vi "PFD_Attitude.vi"(8 "Refresh Rate (Hz)":u32=60) -> ()   [LabVIEW 2023]
uses:
  <vilib>/Utility/miscctls.llb/LVBoundsTypeDef.ctl
  PFD_global.vi
panel:
  in  "Draw Area Size":T1={"Width"=500, "Height"=500}
  in  "att_center":cluster{"y":i16, "y":i16}={"y"=250, "y"=250}
  out "att_pitch":i16
  out "att_roll":i16
  out "x .or. y?":bool
  out "PFD_AttitudeControl":cluster{"Roll":sgl, "Pitch":sgl}
  out "PFD_Attitude":picture
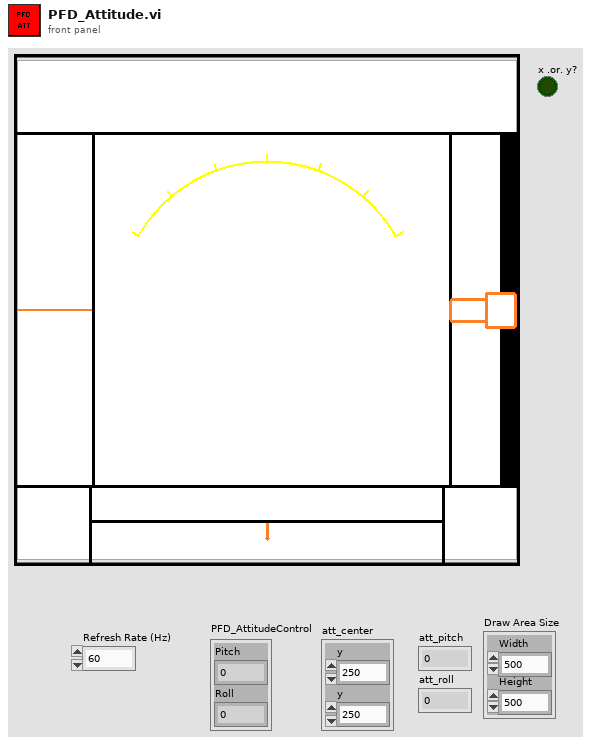
[diagram p1: front panel]
types:
  T1 = typedef "LVBoundsTypeDef.ctl" = cluster{"Width":u32, "Height":u32}
  T2 = cluster{"left":i16, "top":i16, "right":i16, "bottom":i16}
  T3 = cluster{"Width":u16, "Style":enum32{"Solid", "Dash", "Dot", "DashDot", "DashDotDot"}}
  T4 = cluster{"Font Name:":string, "Size":i16, "Strikeout?":bool, "Italic?":bool, "Underline?":bool, "Outline?":bool, "Shadow?":bool, "Bold?":bool}
  T5 = enum16{"User-specified Font", "Application Font", "System Font", "Dialog Font"}
  T6 = cluster{"horizontal":enum16{"left", "center", "right"}, "vertical":enum16{"top", "center", "bottom"}}
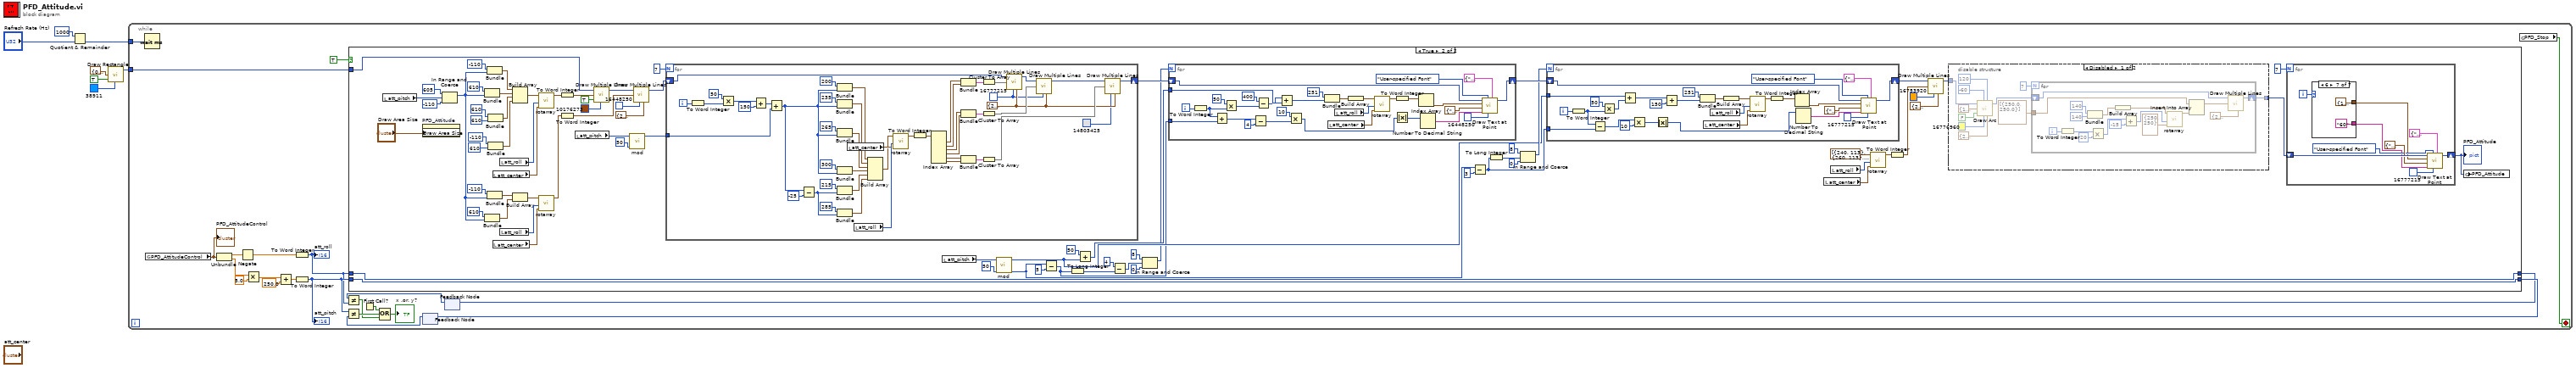
[diagram p0: block diagram]
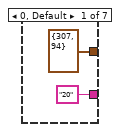
[diagram p3: hidden frame]
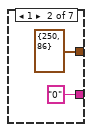
[diagram p4: hidden frame]
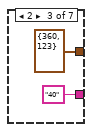
[diagram p5: hidden frame]
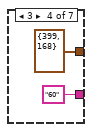
[diagram p6: hidden frame]
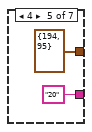
[diagram p7: hidden frame]
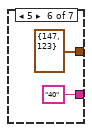
[diagram p8: hidden frame]
diagram:
  n1 = Quotient & Remainder(x=u32 1000, y="Refresh Rate (Hz)") -> (floor(x/y)=w2:u32)  [unwired: 1 out]
  n2 = call <vilib>:"Draw Rectangle.vi"("rect"=T2 {"left"=0, "top"=0, "right"=500, "bottom"=500}, "fill?(F)"=TRUE, "color(black)"=u32 38911 ("Air Color")) -> ("new picture"=w5:picture)  [unwired: 6 in]
  n3 = while {
    tunnel: w5 -> [w29]
    tunnel: w2 -> [w17]
    stop <- w8 stop-if-true
    n4 = Wait (ms)(milliseconds to wait=w17) -> ()  [unwired: 1 out]
    n5 = global read "PFD_global.vi" "PFD_AttitudeControl"() -> (w16:cluster{"Roll":sgl, "Pitch":sgl})
    "PFD_AttitudeControl" <- w16
    n6 = Unbundle(w16) -> ("Roll"=w15:sgl, "Pitch"=w27:sgl)
    n7 = Negate(x=w15) -> (-x=w14:sgl)
    n8 = Multiply(x=w27, y=sgl 5.0) -> (x*y=w13:sgl)
    n9 = Add(x=w13, y=sgl 250.0) -> (x+y=w25:sgl)
    n10 = To Word Integer(number=w14) -> (16bit integer=w11:i16)
    "att_roll" <- w11
    n11 = To Word Integer(number=w25) -> (16bit integer=w12:i16)
    "att_pitch" <- w12
    n12 = case shown="True" TRUE {
      tunnel: w29 -> [_ w107]
      tunnel: w11 -> [w30 w101]
      tunnel: w12 -> [w31 w102]
      tunnel: [w31 w102] -> w23
      tunnel: [w30 w101] -> w20
      frame False {
      }
      frame True {
        n13 = local read "att_pitch"() -> (w76:i16)
        n14 = property on="PFD_Attitude" class="Pict"("Draw Area Size"="Draw Area Size") -> ()  [unwired: 2 in, 2 out]
        n15 = In Range and Coerce(upper limit=i16 605, x=w76, lower limit=i16 -110) -> (coerced(x)=w73:i16)  [unwired: 1 out]
        n16 = Bundle(i16 610, "upper limit"=w73) -> (w64:cluster{i16, "upper limit":i16})  [unwired: 1 in]
        n17 = Bundle(i16 610, "upper limit"=w73) -> (w54:cluster{i16, "upper limit":i16})  [unwired: 1 in]
        n18 = Bundle(i16 -110, "upper limit"=w73) -> (w63:cluster{i16, "upper limit":i16})  [unwired: 1 in]
        n19 = Bundle(i16 -110, "upper limit"=w73) -> (w53:cluster{i16, "upper limit":i16})  [unwired: 1 in]
        n20 = Bundle(i16 610, i16 610) -> (w65:cluster{i16, i16})  [unwired: 1 in]
        n21 = Bundle(i16 -110, i16 610) -> (w66:cluster{i16, i16})  [unwired: 1 in]
        n22 = local read "att_center"() -> (w68:cluster{"y":i16, "y":i16})
        n23 = local read "att_center"() -> (w52:cluster{"y":i16, "y":i16})
        n24 = local read "att_roll"() -> (w67:i16)
        n25 = local read "att_roll"() -> (w51:i16)
        n26 = Build Array(w63, w64, w65, w66) -> (w56:cluster{i16, "upper limit":i16}[])
        n27 = Build Array(w53, w54) -> (w55:cluster{i16, "upper limit":i16}[])
        n28 = call "rotarray.vi"("Pixel Center"=w68, "Angle"=w67, "Array in"=w56) -> ("Array out"=w71:cluster{dbl, dbl}[])  [unwired: 8 in]
        n29 = call "rotarray.vi"("Pixel Center"=w52, "Angle"=w51, "Array in"=w55) -> ("Array out"=w47:cluster{dbl, dbl}[])  [unwired: 8 in]
        n30 = To Word Integer(number=w71) -> (16bit integer=w72:cluster{i16, i16}[])
        n31 = To Word Integer(number=w47) -> (16bit integer=w48:cluster{i16, i16}[])
        n32 = local read "att_pitch"() -> (w78:i16)
        n33 = call <vilib>:"Draw Multiple Lines.vi"("picture"=w107, "line endpoints"=w72, "fill?(F)"=TRUE, "color(black)"=u32 10176273 ("Ground Color")) -> ("new picture"=w46:picture)  [unwired: 5 in]
        n34 = call "mod.vi"("Divide"=i16 50, "Value In"=w78) -> ("Value out"=w104:i16)  [unwired: 8 in, 1 out]
        n35 = call <vilib>:"Draw Multiple Lines.vi"("picture"=w46, "line endpoints"=w48, "color(black)"=u32 16448250, "pen"=T3 {"Width"=2, "Style"=enum."Solid"}) -> ("new picture"=w77:picture)  [unwired: 5 in]
        n36 = for {
          N: 7 ("Numeric") -> [_]
          shift-right: [w239] -> w103
          shift-left: w77 -> [w263]
          tunnel: w104 -> [w251]
          i -> [w259]
          w237 = u32 16777215 ("color(black)")
          w245 = T3 {"Width"=2, "Style"=enum."Solid"} ("pen")
          n37 = To Word Integer(number=w259) -> (16bit integer=w255:i16)
          n38 = Multiply(x=i16 50, y=w255) -> (x*y=w219:i16)
          n39 = Add(x=w219, y=i16 150) -> (x+y=w218:i16)
          n40 = Add(x=w218, y=w251) -> (x+y=w243:i16)
          n41 = Subtract(x=w243, y=i16 -25 ("y 2")) -> (x-y=w241:i16)
          n42 = Bundle(i16 200, w243) -> (w227:cluster{i16, i16})  [unwired: 1 in]
          n43 = Bundle(i16 235, w243) -> (w226:cluster{i16, i16})  [unwired: 1 in]
          n44 = Bundle(i16 265, w243) -> (w225:cluster{i16, i16})  [unwired: 1 in]
          n45 = Bundle(i16 300, w243) -> (w224:cluster{i16, i16})  [unwired: 1 in]
          n46 = Bundle("Numeric 2"=i16 215, w241) -> (w223:cluster{"Numeric 2":i16, i16})  [unwired: 1 in]
          n47 = Bundle("Numeric 3"=i16 285, w241) -> (w222:cluster{"Numeric 3":i16, i16})  [unwired: 1 in]
          n48 = local read "att_center"() -> (w235:cluster{"y":i16, "y":i16})
          n49 = local read "att_roll"() -> (w236:i16)
          n50 = Build Array(w227, w226, w225, w224, w223, w222) -> (w221:cluster{"Numeric 3":i16, i16}[])
          n51 = call "rotarray.vi"("Pixel Center"=w235, "Angle"=w236, "Array in"=w221) -> ("Array out"=w252:cluster{dbl, dbl}[])  [unwired: 8 in]
          n52 = To Word Integer(number=w252) -> (16bit integer=w234:cluster{i16, i16}[])
          n53 = Index Array(array=w234) -> (element #1=w233:cluster{i16, i16}, element #2=w232:cluster{i16, i16}, element #3=w231:cluster{i16, i16}, element #4=w230:cluster{i16, i16}, element #5=w229:cluster{i16, i16}, element #6=w228:cluster{i16, i16})  [unwired: 6 in]
          n54 = Bundle(w233, w232) -> (w250:cluster{cluster{i16, i16}, cluster{i16, i16}})  [unwired: 1 in]
          n55 = Bundle(w231, w230) -> (w249:cluster{cluster{i16, i16}, cluster{i16, i16}})  [unwired: 1 in]
          n56 = Bundle(w229, w228) -> (w238:cluster{cluster{i16, i16}, cluster{i16, i16}})  [unwired: 1 in]
          n57 = Cluster To Array(cluster=w250) -> (array=w254:cluster{i16, i16}[])
          n58 = Cluster To Array(cluster=w249) -> (array=w253:cluster{i16, i16}[])
          n59 = Cluster To Array(cluster=w238) -> (array=w246:cluster{i16, i16}[])
          n60 = call <vilib>:"Draw Multiple Lines.vi"("picture"=w263, "line endpoints"=w254, "color(black)"=w237, "pen"=w245) -> ("new picture"=w256:picture)  [unwired: 5 in]
          n61 = call <vilib>:"Draw Multiple Lines.vi"("picture"=w256, "line endpoints"=w253, "color(black)"=w237, "pen"=w245) -> ("new picture"=w247:picture)  [unwired: 5 in]
          n62 = call <vilib>:"Draw Multiple Lines.vi"("picture"=w247, "line endpoints"=w246, "color(black)"=u32 14803425, "pen"=w245) -> ("new picture"=w239:picture)  [unwired: 5 in]
        }
        n63 = local read "att_pitch"() -> (w94:i16)
        n64 = call "mod.vi"("Divide"=i16 50, "Value In"=w94) -> ("Ceil"=w81:i16, "Value out"=w91:i16)  [unwired: 8 in]
        n65 = Subtract(x=w81, y=i16 5) -> (x-y=w82:i16)
        n66 = To Long Integer(number=w82) -> (32bit integer=w83:i32)
        n67 = Add(x=i16 50 ("y"), y=w91) -> (x+y=w90:i16)
        n68 = Subtract(x=4 ("Numeric"), y=w83) -> (x-y=w85:i32)
        n69 = In Range and Coerce(upper limit=8, x=w85, lower limit=0) -> (coerced(x)=w84:i32)  [unwired: 1 out]
        n70 = for {
          N: w84 -> [_]
          shift-right: [w205] -> w100
          shift-left: w103 -> [w207]
          tunnel: w90 -> [w198]
          tunnel: w82 -> [w191]
          i -> [w201]
          n71 = To Word Integer(number=w201) -> (16bit integer=w192:i16)
          n72 = Add(x=w192, y=w191) -> (x+y=w190:i16)
          n73 = Multiply(x=i16 50, y=w192) -> (x*y=w197:i16)
          n74 = Subtract(x=w190, y=i16 4 ("y 2")) -> (x-y=w188:i16)
          n75 = Subtract(x=i16 400 ("y 4"), y=w197) -> (x-y=w196:i16)
          n76 = Add(x=w196, y=w198) -> (x+y=w195:i16)
          n77 = Multiply(x=i16 10, y=w188) -> (x*y=w193:i16)
          n78 = Bundle("Numeric 2"=i16 251, w195) -> (w212:cluster{"Numeric 2":i16, i16})  [unwired: 1 in]
          n79 = local read "att_center"() -> (w203:cluster{"y":i16, "y":i16})
          n80 = local read "att_roll"() -> (w206:i16)
          n81 = Build Array(w212) -> (w211:cluster{"Numeric 2":i16, i16}[])
          n82 = call "rotarray.vi"("Pixel Center"=w203, "Angle"=w206, "Array in"=w211) -> ("Array out"=w209:cluster{dbl, dbl}[])  [unwired: 8 in]
          n83 = To Word Integer(number=w209) -> (16bit integer=w208:cluster{i16, i16}[])
          n84 = Absolute Value(x=w193) -> (abs(x)=w202:i16)
          n85 = Index Array(array=w208) -> (element=w210:cluster{i16, i16})  [unwired: 1 in]
          n86 = Number To Decimal String(number=w202) -> (decimal integer string=w214:string)  [unwired: 1 in]
          n87 = call <vilib>:"Draw Text at Point.vi"("[user-specified font]"=T4 {"Font Name:"="a", "Size"=18, "Strikeout?"=FALSE, "Italic?"=FALSE, "Underline?"=FALSE, "Outline?"=FALSE, "Shadow?"=FALSE, "Bold?"=TRUE}, "text color(black)"=u32 16448250, "desired font(Application)"=T5."User-specified Font", "text"=w214, "alignment(left, top)"=T6 {"horizontal"=enum."center", "vertical"=enum."center"}, "origin"=w210, "picture"=w207) -> ("new picture"=w205:picture)  [unwired: 3 in, 1 out]
        }
        n88 = Subtract(x=w81, y=i16 3) -> (x-y=w80:i16)
        n89 = To Long Integer(number=w80) -> (32bit integer=w98:i32)
        n90 = In Range and Coerce(upper limit=8, x=w98, lower limit=0) -> (coerced(x)=w95:i32)  [unwired: 1 out]
        n91 = for {
          N: w95 -> [_]
          shift-right: [w173] -> w33
          shift-left: w100 -> [w172]
          tunnel: w91 -> [w168]
          tunnel: w80 -> [w160]
          i -> [w185]
          n92 = To Word Integer(number=w185) -> (16bit integer=w161:i16)
          n93 = Subtract(x=w161, y=w160) -> (x-y=w163:i16)
          n94 = Multiply(x=i16 50, y=w161) -> (x*y=w183:i16)
          n95 = Add(x=w168, y=w183) -> (x+y=w167:i16)
          n96 = Multiply(x=w163, y=i16 10) -> (x*y=w162:i16)
          n97 = Absolute Value(x=w162) -> (abs(x)=w187:i16)
          n98 = Add(x=w167, y=i16 150) -> (x+y=w165:i16)
          n99 = Bundle("Numeric 2"=i16 251, w165) -> (w178:cluster{"Numeric 2":i16, i16})  [unwired: 1 in]
          n100 = local read "att_center"() -> (w169:cluster{"y":i16, "y":i16})
          n101 = local read "att_roll"() -> (w171:i16)
          n102 = Build Array(w178) -> (w177:cluster{"Numeric 2":i16, i16}[])
          n103 = call "rotarray.vi"("Pixel Center"=w169, "Angle"=w171, "Array in"=w177) -> ("Array out"=w175:cluster{dbl, dbl}[])  [unwired: 8 in]
          n104 = To Word Integer(number=w175) -> (16bit integer=w176:cluster{i16, i16}[])
          n105 = Index Array(array=w176) -> (element=w174:cluster{i16, i16})  [unwired: 1 in]
          n106 = Number To Decimal String(number=w187) -> (decimal integer string=w186:string)  [unwired: 1 in]
          n107 = call <vilib>:"Draw Text at Point.vi"("[user-specified font]"=T4 {"Font Name:"="a", "Size"=18, "Strikeout?"=FALSE, "Italic?"=FALSE, "Underline?"=FALSE, "Outline?"=FALSE, "Shadow?"=FALSE, "Bold?"=TRUE}, "text color(black)"=u32 16777215, "desired font(Application)"=T5."User-specified Font", "text"=w186, "alignment(left, top)"=T6 {"horizontal"=enum."center", "vertical"=enum."center"}, "origin"=w174, "picture"=w172) -> ("new picture"=w173:picture)  [unwired: 3 in, 1 out]
        }
        n108 = local read "att_center"() -> (w37:cluster{"y":i16, "y":i16})
        n109 = local read "att_roll"() -> (w36:i16)
        n110 = call "rotarray.vi"("Pixel Center"=w37, "Angle"=w36, "Array in"=cluster{"x":i16, "y":i16}[] [{"x"=240, "y"=113}, {"x"=260, "y"=113}, {"x"=250, "y"=103}, {"x"=240, "y"=113}] ("line endpoints")) -> ("Array out"=w34:cluster{dbl, dbl}[])  [unwired: 8 in]
        n111 = To Word Integer(number=w34) -> (16bit integer=w39:cluster{i16, i16}[])
        n112 = call <vilib>:"Draw Multiple Lines.vi"("picture"=w33, "line endpoints"=w39, "color(black)"=u32 16753920, "pen"=T3 {"Width"=2, "Style"=enum."Solid"}) -> ("new picture"=w32:picture)  [unwired: 5 in]
        n113 = disable-structure shown="Disabled" {
          disable-tunnel: w32 -> [w131 w159]
          disable-tunnel: [w133 w159] -> w43
          frame Disabled {
            n114 = call <vilib>:"Draw Arc.vi"("picture"=w131, "start angle[degrees]"=i16 -60, "rect"=T2 {"left"=100, "top"=100, "right"=400, "bottom"=400}, "fill?(F)"=FALSE, "color(black)"=u32 16776960, "arc size[degrees]"=i16 120, "pen"=T3 {"Width"=2, "Style"=enum."Solid"}) -> ("new picture"=w132:picture)  [unwired: 2 in]
            n115 = for {
              N: 7 ("Numeric") -> [_]
              shift-right: [w157] -> w133
              shift-left: w132 -> [w156]
              tunnel: cluster{dbl, dbl}[] [{250.0, 250.0}] ("Array") -> [w145]
              i -> [w151]
              n116 = To Word Integer(number=w151) -> (16bit integer=w150:i16)
              n117 = Bundle("y 2"=i16 140, "y 3"=i16 140) -> (w153:cluster{"y 2":i16, "y 3":i16})  [unwired: 1 in]
              n118 = Multiply(x=w150, y=i16 20) -> (x*y=w147:i16)
              n119 = Build Array(w153) -> (w152:cluster{"y 2":i16, "y 3":i16}[])
              n120 = Add(x=w147, y=i16 -15) -> (x+y=w146:i16)
              n121 = call "rotarray.vi"("Pixel Center"=cluster{i16, i16} {250, 250}, "Angle"=w146, "Array in"=w152) -> ("Array out"=w144:cluster{dbl, dbl}[])  [unwired: 8 in]
              n122 = Insert Into Array(array=w145, new element=w144) -> (w143:cluster{dbl, dbl}[])  [unwired: 1 in]
              n123 = call <vilib>:"Draw Multiple Lines.vi"("picture"=w156, "line endpoints"=w143, "pen"=T3 {"Width"=2, "Style"=enum."Solid"}) -> ("new picture"=w157:picture)  [unwired: 6 in]
            }
          }
          frame Enabled {
          }
        }
        n124 = for {
          N: 7 ("Numeric") -> [_]
          shift-right: [w115] -> w42
          shift-left: w43 -> [w116]
          i -> [w111]
          n125 = case shown="6" w111 {
            tunnel: ["20" ("text 2") "0" ("text") "40" ("text") "60" ("text") "20" ("text") "40" ("text") "60" ("text")] -> w110
            tunnel: [cluster{"x":i16, "y":i16} {"x"=307, "y"=94} ("origin 2") cluster{"x":i16, "y":i16} {"x"=250, "y"=86} ("origin") cluster{"x":i16, "y":i16} {"x"=360, "y"=123} ("origin") cluster{"x":i16, "y":i16} {"x"=399, "y"=168} ("origin") cluster{"x":i16, "y":i16} {"x"=194, "y"=95} ("origin") cluster{"x":i16, "y":i16} {"x"=147, "y"=123} ("origin") cluster{"x":i16, "y":i16} {"x"=107, "y"=166} ("origin")] -> w109
            frame 0, Default {
            }
            frame 1 {
            }
            frame 2 {
            }
            frame 3 {
            }
            frame 4 {
            }
            frame 5 {
            }
            frame 6 {
            }
          }
          n126 = call <vilib>:"Draw Text at Point.vi"("[user-specified font]"=T4 {"Font Name:"="a", "Size"=19, "Strikeout?"=FALSE, "Italic?"=FALSE, "Underline?"=FALSE, "Outline?"=FALSE, "Shadow?"=FALSE, "Bold?"=TRUE}, "text color(black)"=u32 16777215, "desired font(Application)"=T5."User-specified Font", "text"=w110, "alignment(left, top)"=T6 {"horizontal"=enum."center", "vertical"=enum."center"}, "origin"=w109, "picture"=w116) -> ("new picture"=w115:picture)  [unwired: 3 in, 1 out]
        }
        "PFD_Attitude" <- w42
        n127 = global write "PFD_global.vi" "PFD_Attitude"(w42) -> ()
      }
    }
    n128 = First Call?() -> (First Call?: T/F=w24:bool)
    n129 = feedback-in #1(w23) -> ()
    n130 = feedback #1() -> (w22:i16)  [unwired: 1 in]
    n131 = Not Equal?(x=w12, y=w22) -> (x != y?=w21:bool)
    n132 = feedback-in #2(w20) -> ()
    n133 = feedback #2() -> (w19:i16)  [unwired: 1 in]
    n134 = Not Equal?(x=w19, y=w11) -> (x != y?=w18:bool)
    n135 = Compound Arithmetic op=OR(w24, w21, w18) -> (→"x .or. y?":bool)
    n136 = global read "PFD_global.vi" "PFD_Stop"() -> (w8:bool)
  }
